vi "tokens to path.vi"(10 "Data Access:OS":T1, 11 "array of strings":string[](array[string])) -> (3 "String":string)   [LabVIEW 2013, in "PL Framework Configuration Tool.lvlib"]
uses:
  PL Framework Configuration Tool.lvlib
  <vilib>/NI/Tag Bus Module Framework/root configuration/Target Types.ctl
  <vilib>/NI/Tag Bus Module Framework/root configuration/TBM configuration.lvclass
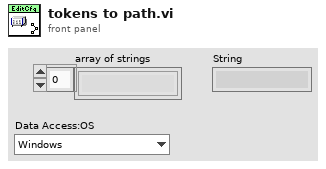
[diagram p1: front panel]
types:
  T1 = typedef "TBM configuration.lvclass/Target Types.ctl" = enum16{"Windows", "Mac", "Linux", "Linux RT ARM", "VxWorks", "Pharlap", "Other", "Linux RT x64"}
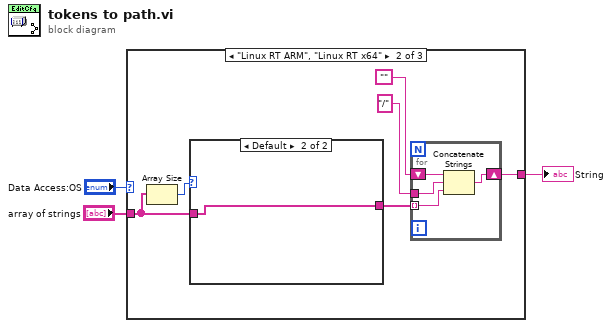
[diagram p0: block diagram]
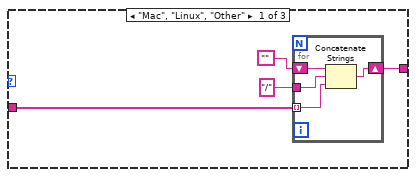
[diagram p2: hidden frame]
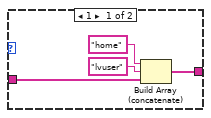
[diagram p3: hidden frame]
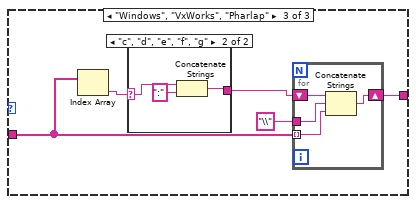
[diagram p4: hidden frame]
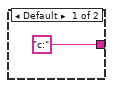
[diagram p5: hidden frame]
diagram:
  n1 = case shown="\"Linux RT ARM\", \"Linux RT x64\"" "Data Access:OS" {
    tunnel: "array of strings" -> [w7 w13 w29]
    tunnel: [w6 w17 w31] -> w3
    frame "Mac", "Linux", "Other" {
      n2 = for {
        tunnel: w7 -> [w10] mode=indexing
        shift-right: [w9] -> w6
        shift-left: "" -> [w11]
        tunnel: "/" -> [w8]
        n3 = Concatenate Strings(w11, w8, w10) -> (w9:string)
      }
    }
    frame "Linux RT ARM", "Linux RT x64" {
      n4 = Array Size(array=w13) -> (size(s)=w12:i32)
      n5 = case shown="Default" w12 {
        tunnel: w13 -> [w21 w22]
        tunnel: [w18 w22] -> w14
        frame 1 {
          n6 = Build Array (concatenate)("home", "lvuser", w21) -> (w18:string[])
        }
        frame Default {
        }
      }
      n7 = for {
        tunnel: w14 -> [w25] mode=indexing
        shift-right: [w24] -> w17
        shift-left: "" -> [w26]
        tunnel: "/" -> [w23]
        n8 = Concatenate Strings(w26, w23, w25) -> (w24:string)
      }
    }
    frame "Windows", "VxWorks", "Pharlap" {
      n9 = Index Array(array=w29) -> (element=w28:string)  [unwired: 1 in]
      n10 = case shown="\"c\", \"d\", \"e\", \"f\", \"g\"" w28 {
        selector: w28 -> [_ w35]
        tunnel: ["c:" w33] -> w27
        frame Default {
        }
        frame "c", "d", "e", "f", "g" {
          n11 = Concatenate Strings(w35, ":" ("string")) -> (w33:string)
        }
      }
      n12 = for {
        tunnel: w29 -> [w38] mode=indexing
        shift-right: [w37] -> w31
        shift-left: w27 -> [w39]
        tunnel: "\\" -> [w36]
        n13 = Concatenate Strings(w39, w36, w38) -> (w37:string)
      }
    }
  }
  "String" <- w3
